vi "sub_Ave_Power_And_Thresholding.vi"(0 "Input Complex Samples":cdb[](array[numeric]), 7 "bin_size":i32, 11 "threshold":dbl) -> (4 "Averaged Power Signal":dbl[](array[numeric]), 8 "Thresholded Signal":bool[](array[boolean]))   [LabVIEW 2023]
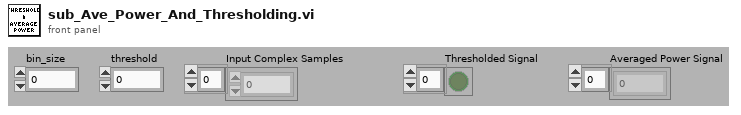
[diagram p1: front panel]
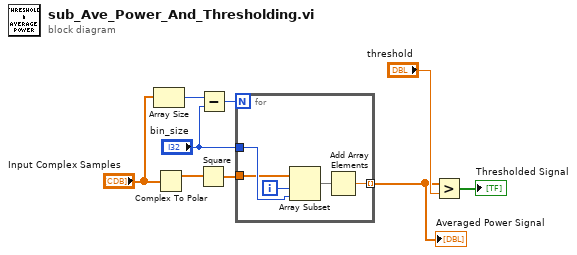
[diagram p0: block diagram]
diagram:
  n1 = Array Size(array="Input Complex Samples") -> (size(s)=w8:i32)
  n2 = Complex To Polar(r * e^(i*theta)="Input Complex Samples") -> (r=w3:dbl[])  [unwired: 1 out]
  n3 = Square(x=w3) -> (x^2=w1:dbl[])
  n4 = Subtract(x=w8, y="bin_size") -> (x-y=w7:i32)
  n5 = for {
    N: w7 -> [_]
    tunnel: "bin_size" -> [w13]
    tunnel: [w11] -> w4 mode=indexing
    tunnel: w1 -> [w10]
    i -> [w12]
    n6 = Array Subset(array=w10, index=w12, length=w13) -> (w14:dbl[])
    n7 = Add Array Elements(numeric array=w14) -> (sum=w11:dbl)
  }
  "Averaged Power Signal" <- w4
  n8 = Greater?(x=w4, y="threshold") -> (0:→"Thresholded Signal":bool[])
